vi "set Zoom Level.vi"(10 "Zoom Level":T1=enum."Close", 11 "Camera in":refnum<class "Camera.lvclass">) -> (3 "Camera out":refnum<class "Camera.lvclass">)   [LabVIEW 2015, in "Camera.lvclass"]
uses:
  Camera.lvclass
  Zoom Level.ctl
  Camera.lvclass/Camera.ctl
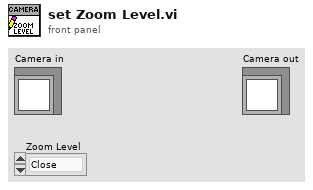
[diagram p1: front panel]
types:
  T1 = typedef "Camera.lvclass/Zoom Level.ctl" = enum16{"Far", "Medium", "Close"}
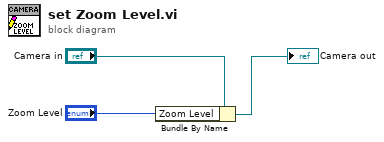
[diagram p0: block diagram]
diagram:
  n1 = Bundle By Name(cluster="Camera in", "Zoom Level"="Zoom Level") -> (→"Camera out":refnum<class "Camera.lvclass">)
